vi "main.vi"() -> ()   [LabVIEW 2017]
uses:
  typeDefs/programControl.ctl
panel:
  in  "stop":bool
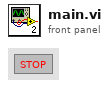
[diagram p1: front panel]
types:
  T1 = typedef "programControl.ctl" = enum16{"init", "run", "end"}
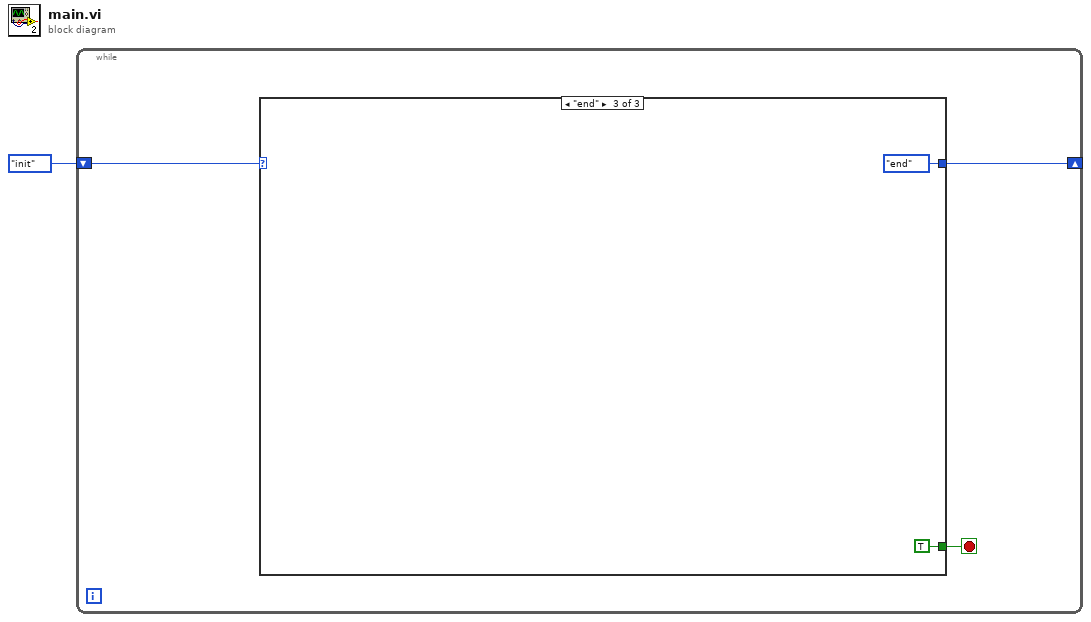
[diagram p0: block diagram]
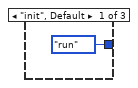
[diagram p2: hidden frame]
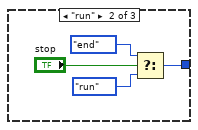
[diagram p3: hidden frame]
diagram:
  n1 = while {
    shift-right: [w3] -> _
    shift-left: programControl."init" -> [w4]
    stop <- w2 stop-if-true
    n2 = case shown="\"end\"" w4 {
      tunnel: [programControl."run" w6 programControl."end"] -> w3
      tunnel: [_ _ TRUE] -> w2
      frame "init", Default {
      }
      frame "run" {
        n3 = Select(t=programControl."end", s="stop", f=programControl."run") -> (s? t:f=w6:T1)
      }
      frame "end" {
      }
    }
  }
